vi "_var to class.vi"(7 "In":refnum<class "Value.lvclass">, 8 "error in":errorcluster, 11 "variant":variant) -> (0 "error out":errorcluster, 2 "valid":bool, 3 "Out":refnum<class "Value.lvclass">)   [LabVIEW 2023, in "LabGRAD.lvlib" / "Value.lvclass"]
uses:
  Value.lvclass
  Value.lvclass/Value.ctl
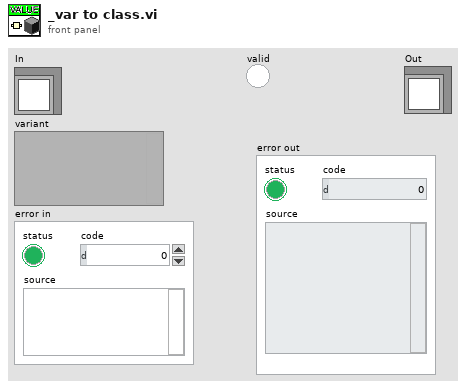
[diagram p1: front panel]
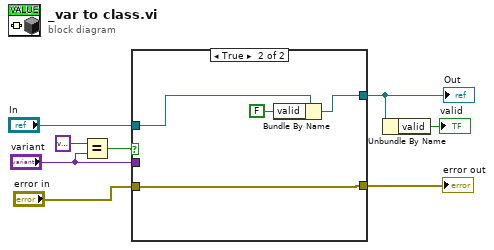
[diagram p0: block diagram]
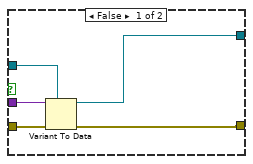
[diagram p2: hidden frame]
diagram:
  n1 = Equal?(x=variant, y="variant") -> (x = y?=w3:bool)
  n2 = case shown="True" w3 {
    tunnel: "variant" -> [w13 _]
    tunnel: "In" -> [w12 w14]
    tunnel: "error in" -> [w11 w17]
    tunnel: [w10 w17] -> w6
    tunnel: [w9 w16] -> w2
    frame False {
      n3 = Variant To Data(error in=w11, type=w12, Variant=w13) -> (data=w9:refnum<class "Value.lvclass">, error out=w10:errorcluster)
    }
    frame True {
      n4 = Bundle By Name(cluster=w14, "valid"=FALSE) -> (w16:refnum<class "Value.lvclass">)
    }
  }
  "error out" <- w6
  "Out" <- w2
  n5 = Unbundle By Name(w2) -> ("valid"=→"valid":bool)
